vi "TTT_main 4.vi"() -> ()   [LabVIEW 8.6]
uses:
  subvi/titati1.ctl
panel:
  in  "instruction":dbl[][](array[numeric]) caption="Hit number key on KB"
  out "Slots":refnum<vi>[](array[refnum])
  out "hit_disp":i32
  out "1p_last":i32[](array[numeric])
  in  "hls 9":bool
  in  "hls 8":bool
  in  "hls 7":bool
  in  "hls 6":bool
  in  "hls 5":bool
  in  "hls 4":bool
  in  "hls 3":bool
  in  "hls 2":bool
  in  "hls":bool
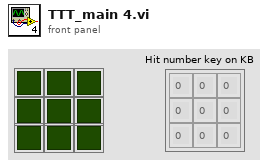
[diagram p1: front panel]
types:
  T1 = typedef "titati1.ctl" = enum16{"Init", "idle", "1P", "CPU", "end"}
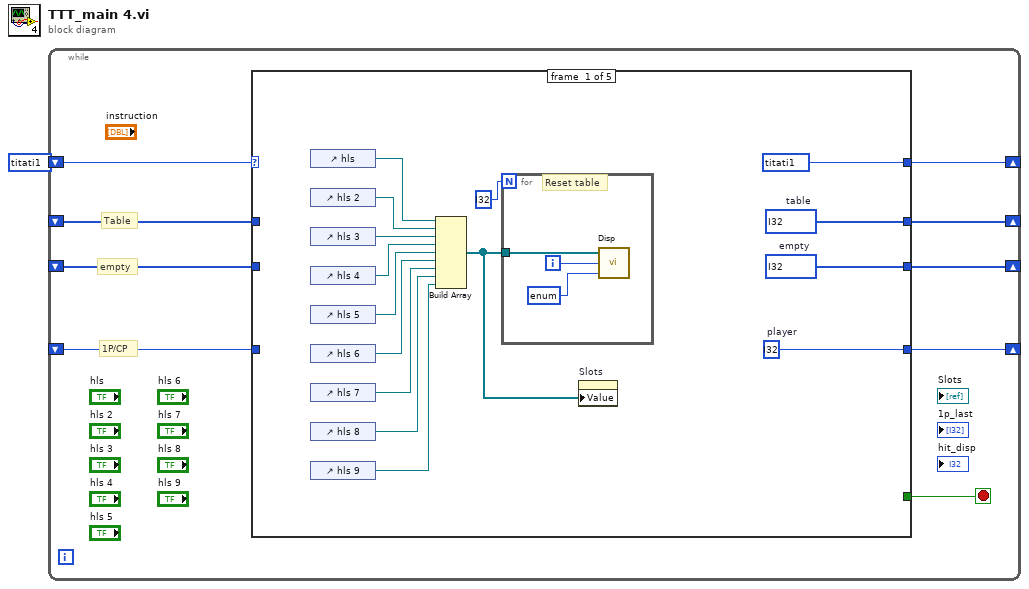
[diagram p0: block diagram]
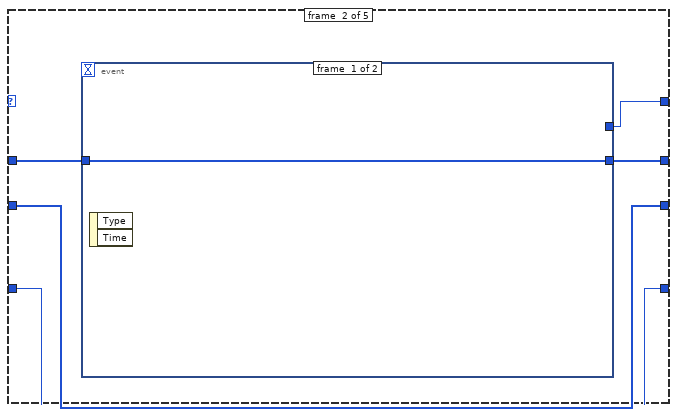
[diagram p2: hidden frame]
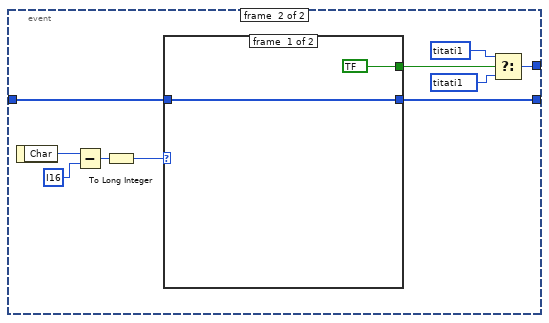
[diagram p3: hidden frame]
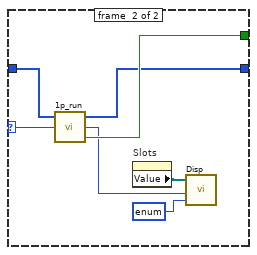
[diagram p4: hidden frame]
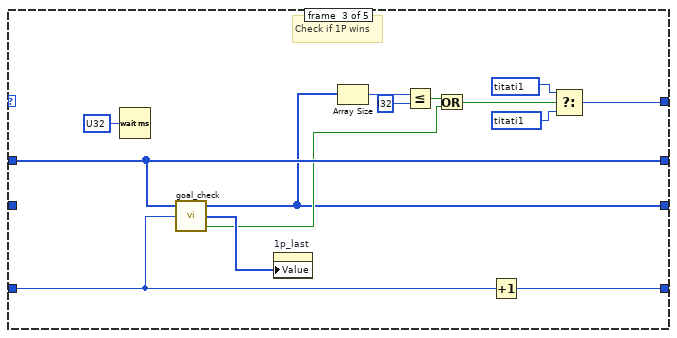
[diagram p5: hidden frame]
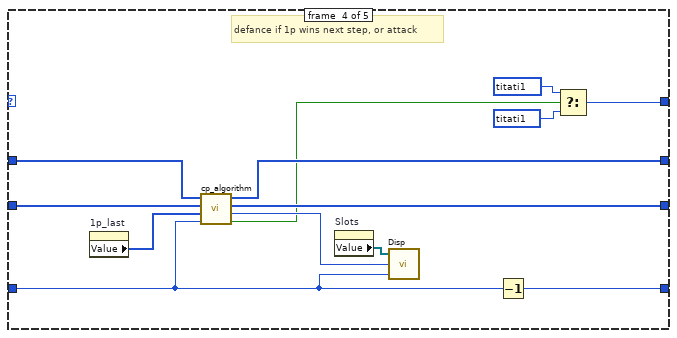
[diagram p6: hidden frame]
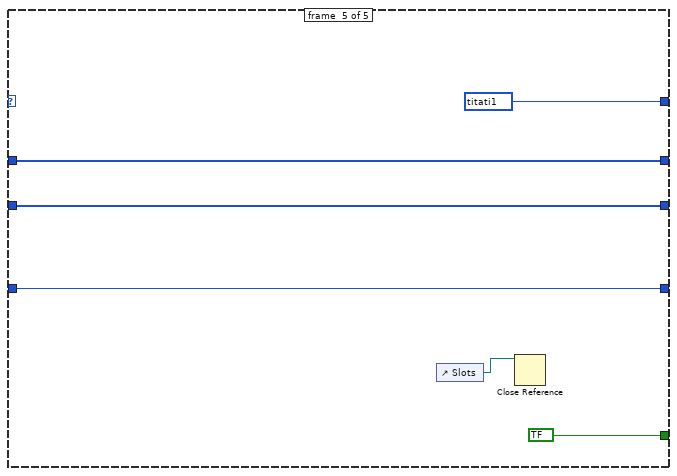
[diagram p7: hidden frame]
diagram:
  n1 = while {
    shift-right: [w8] -> _
    shift-left: T1 ? ("Actoion") -> [w10]
    shift-right: [w6] -> _
    shift-left: _ -> [w7]
    shift-right: [w4] -> _
    shift-left: _ -> [w2]
    shift-right: [w3] -> _
    shift-left: _ -> [w5]
    stop <- w9 stop-if-true
    # "empty"
    # "Table"
    # "1P/CP"
    n2 = case shown="\"end\"" w10 {
      tunnel: [_ _ _ _ bool ?] -> w9
      tunnel: [T1 ? ("Actoion") w33 w64 w76 T1 ? ("Actoion")] -> w8
      tunnel: w7 -> [_ w32 w62 w75 w81]
      tunnel: [w13 w32 w67 w80 w81] -> w6
      tunnel: w5 -> [_ w29 _ w72 w83]
      tunnel: [w12 w30 w60 w70 w84] -> w4
      tunnel: [w11 w29 w54 w69 w83] -> w3
      tunnel: w2 -> [_ w31 w60 w71 w84]
      frame #0 {
        w11 = i32[] ?  # empty
        w13 = i32 ?  # player
        w12 = i32[] ?  # table
        n3 = control-ref of="hls"() -> (w25:refnum<vi>)
        n4 = control-ref of="hls 2"() -> (w24:refnum<vi>)
        n5 = control-ref of="hls 3"() -> (w23:refnum<vi>)
        n6 = control-ref of="hls 4"() -> (w22:refnum<vi>)
        n7 = control-ref of="hls 5"() -> (w21:refnum<vi>)
        n8 = control-ref of="hls 6"() -> (w20:refnum<vi>)
        n9 = control-ref of="hls 7"() -> (w19:refnum<vi>)
        n10 = control-ref of="hls 8"() -> (w18:refnum<vi>)
        n11 = control-ref of="hls 9"() -> (w17:refnum<vi>)
        n12 = Build Array(w25, w24, w23, w22, w21, w20, w19, w18, w17) -> (w14:refnum<vi>[])
        n13 = for {
          N: i32 ? -> [_]
          tunnel: w14 -> [w28]
          i -> [w26]
          # "Reset table"
          n14 = call "Disp.vi"("Slot_color"=enum16{"0", "1", "2"} ?, "index"=w26, "Slot"=w28) -> ()  [unwired: 3 in]
        }
        n15 = property on="Slots" class="Arr (strict)"("Value"=w14) -> ()  [unwired: 2 in, 2 out]
      }
      frame #1 {
        n16 = event shown="[1] Key Down" {
          selector: _ -> [_ _]
          dyn-events: _ -> [_ _]
          timeout: _ -> [_ _]
          tunnel: [_ w42] -> w33
          tunnel: w31 -> [w34 w40]
          tunnel: [w34 w39] -> w30
          event #0 {
            n17 = event-data() -> ()  [unwired: 1 in, 2 out]
          }
          event #1 {
            n18 = event-data() -> ("Char"=w38:i16)  [unwired: 1 in]
            n19 = Subtract(x=w38, y=i16 ?) -> (x-y=w36:i16)
            n20 = To Long Integer(number=w36) -> (32bit integer=w35:i32)
            n21 = case shown="0..8" w35 {
              selector: w35 -> [_ w52]
              tunnel: [bool ? ("no error") w53] -> w41
              tunnel: w40 -> [w45 w48]
              tunnel: [w45 w47] -> w39
              frame #0 {
              }
              frame #1 {
                n22 = call "1p_run.vi"("hit_ind"=w52, "table"=w48) -> ("no error"=w53:bool, "hit_disp"=w49:i32, "table out"=w47:i32[])  [unwired: 1 in]
                n23 = property on="Slots" class="Arr (strict)"() -> ("Value"=w50:refnum<vi>[])  [unwired: 2 in, 2 out]
                n24 = call "Disp.vi"("Slot_color"=enum16{"0", "1", "2"} ?, "index"=w49, "Slot"=w50) -> ()  [unwired: 3 in]
              }
            }
            n25 = Select(t=T1 ? ("Actoion"), s=w41, f=T1 ? ("Actoion")) -> (s? t:f=w42:T1)
          }
        }
      }
      frame #2 {
        # "Check if 1P wins"
        n26 = Wait (ms)(milliseconds to wait=u32 ?) -> ()  [unwired: 1 out]
        n27 = call "goal_check.vi"("flag"=w62, "table"=w60) -> ("fin"=w55:bool, "win step"=w63:i32[], "empty"=w54:i32[])  [unwired: 1 in]
        n28 = property on="1p_last" class="Arr (strict)"("Value"=w63) -> ()  [unwired: 2 in, 2 out]
        n29 = Array Size(array=w54) -> (size(s)=w59:i32)
        n30 = Less Or Equal?(x=w59, y=i32 ?) -> (x <= y?=w57:bool)
        n31 = Or(x=w57, y=w55) -> (x .or. y?=w56:bool)
        n32 = Increment(x=w62) -> (x+1=w67:i32)
        n33 = Select(t=T1 ? ("Actoion"), s=w56, f=T1 ? ("Actoion")) -> (s? t:f=w64:T1)
      }
      frame #3 {
        # "defance if 1p wins next step, or attack"
        n34 = property on="1p_last" class="Arr (strict)"() -> ("Value"=w79:i32[])  [unwired: 2 in, 2 out]
        n35 = call "cp_algorithm.vi"("CP flag"=w75, "1P last"=w79, "empty"=w72, "table"=w71) -> ("CP_fin"=w68:bool, "hit"=w74:i32, "empty out"=w69:i32[], "table out"=w70:i32[])
        n36 = property on="Slots" class="Arr (strict)"() -> ("Value"=w73:refnum<vi>[])  [unwired: 2 in, 2 out]
        n37 = call "Disp.vi"("Slot_color"=w75, "index"=w74, "Slot"=w73) -> ()  [unwired: 3 in]
        n38 = Decrement(x=w75) -> (x-1=w80:i32)
        n39 = Select(t=T1 ? ("Actoion"), s=w68, f=T1 ? ("Actoion")) -> (s? t:f=w76:T1)
      }
      frame #4 {
        n40 = control-ref of="Slots"() -> (w82:refnum<vi>)
        n41 = Close Reference(reference=w82) -> ()  [unwired: 1 in, 1 out]
      }
    }
  }
